vi "CSV - Add New Columns.vi"(8 "error in (no error)":errorcluster, 9 "LV Data Types":T1[](array[typedef]) format="%.0x", 10 "Headers":string[](array[string]), 11 "TableLogger_CSV_Actor in":refnum<class "TableLogger_CSV_Actor.lvclass">) -> (0 "error out":errorcluster, 3 "TableLogger_CSV_Actor out":refnum<class "TableLogger_CSV_Actor.lvclass">)   [LabVIEW 2014, in "TableLogger_CSV_Actor.lvlib" / "TableLogger_CSV_Actor.lvclass"]
uses:
  TableLogger_CSV_Actor.lvclass
  <userlib>/_OpenG.lib/lvdata/lvdata.llb/Type Descriptor Enumeration__ogtk.ctl
  TableLogger_CSV_Actor.lvclass/TableLogger_CSV_Actor.ctl
panel:
  # "Connector Pane"
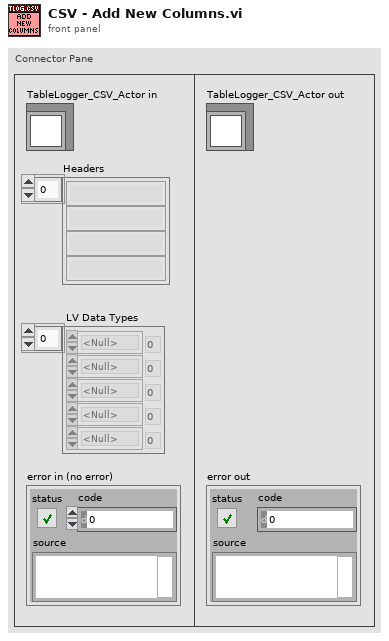
[diagram p1: front panel]
types:
  T1 = typedef "Type Descriptor Enumeration__ogtk.ctl" = enum8{"<Null>", "I8", "I16", "I32", "I64", "U8", "U16", "U32", "U64", "SGL", "DBL", "EXT", "CSG", "CDB", "CXT", "0x0F", "0x10", "0x11", "0x12", "0x13", "0x14", "Enum U8", "Enum U16", "Enum U32", "Enum U64", "SGL PQ", "DBL PQ", "EXT PQ", "CSG PQ", "CDB PQ", "CXT PQ", "0x1F", "0x20", "Boolean", "0x22", "0x23", "0x24", "0x25", "0x26", "0x27", "0x28", "0x29", "0x2A", "0x2B", "0x2C", "0x2D", "0x2E", "0x2F", "String", "0x31", "Path", "Pict", "0x34", "0x35", "0x36", "DAQ", "0x38", "0x39", "0x3A", "0x3B", "0x3C", "0x3D", "0x3E", "0x3F", "Array", "0x41", "0x42", "0x43", "0x44", "0x45", "0x46", "0x47", "0x48", "0x49", "0x4A", "0x4B", "0x4C", "0x4D", "0x4E", "0x4F", "Cluster", "0x51", "0x52", "Variant", "Waveform", "0x55", "0x56", "0x57", "0x58", "0x59", "0x5A", "0x5B", "0x5C", "0x5D", "0x5E", "0x5F", "0x60", "0x61", "0x62", "0x63", "0x64", "0x65", "0x66", "0x67", "0x68", "0x69", "0x6A", "0x6B", "0x6C", "0x6D", "0x6E", "0x6F", "Refnum"}
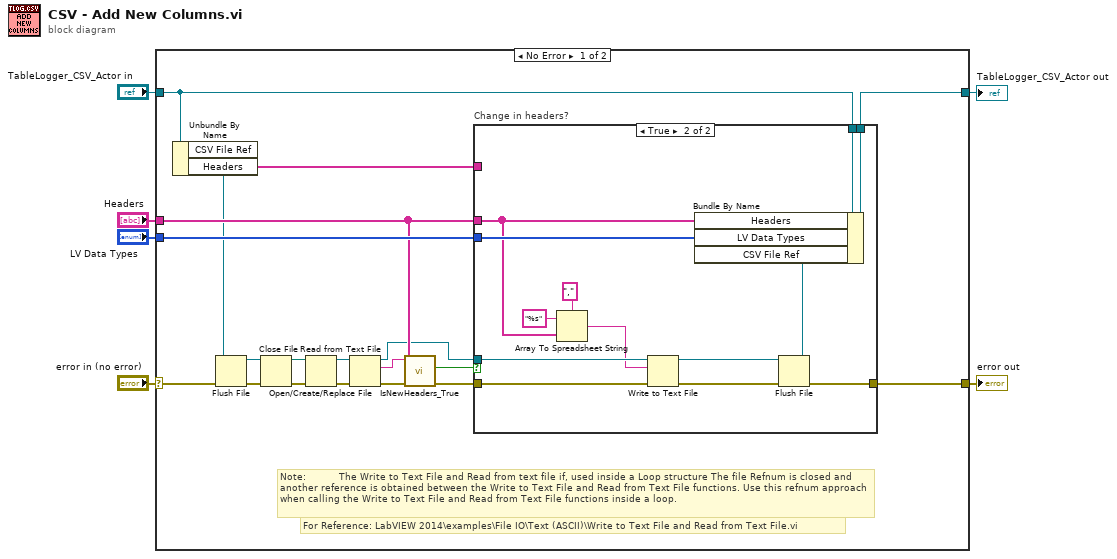
[diagram p0: block diagram]
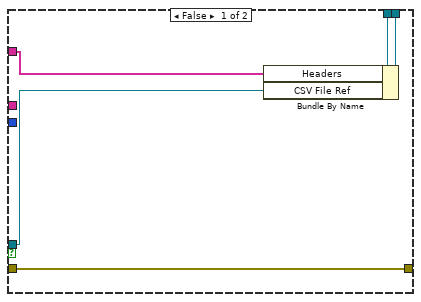
[diagram p2: hidden frame]
diagram:
  n1 = case shown="No Error" "error in (no error)" {
    selector: "error in (no error)" -> [w21 w44]
    tunnel: [w25 w45] -> w6
    tunnel: "Headers" -> [w19 _]
    tunnel: "LV Data Types" -> [w22 _]
    tunnel: [w23 w44] -> w2
    tunnel: "TableLogger_CSV_Actor in" -> [w24 w45]
    frame No Error {
      # "For Reference: LabVIEW 2014\\examples\\File IO\\Text (ASCII)\\Write to Text File and Read from Text File.vi"
      # "Note:           The Write to Text File and Read from text file if, used inside a Loop structure The file Refnum is closed and another reference is obtained between the Write to Text File and Read from Text File functions. Use this refnum approach when calling the Write to Text File and Read from Text File functions inside a loop."
      n2 = Unbundle By Name(w24) -> ("CSV File Ref"=w18:refnum<file>, "Headers"=w8:string[])
      n3 = Flush File(refnum=w18, error in=w21) -> (refnum out=w12:refnum<file>, error out=w10:errorcluster)
      n4 = Close File(refnum=w12, error in=w10) -> (path=w14:path, error out=w13:errorcluster)
      n5 = Open/Create/Replace File(file path (use dialog)=w14, error in=w13) -> (refnum out=w11:refnum<file>, error out=w9:errorcluster)  [unwired: 4 in, 1 out]
      n6 = Read from Text File(file (use dialog)=w11, error in=w9) -> (refnum out=w15:refnum<file>, text=w7:string, error out=w17:errorcluster)  [unwired: 2 in, 1 out]
      n7 = call "IsNewHeaders_True.vi"("error in"=w17, "Headers"=w19, "Data"=w7) -> ("error out"=w16:errorcluster, "Different Header?"=w20:bool)  [unwired: 6 in, 1 out]
      n8 = case "Change in headers?" shown="True" w20 {
        tunnel: [w28 w43] -> w25
        tunnel: w24 -> [w29 w42]
        tunnel: w16 -> [w30 w35]
        tunnel: [w30 w38] -> w23
        tunnel: w22 -> [_ w41]
        tunnel: w19 -> [_ w34]
        tunnel: w15 -> [w27 w36]
        tunnel: w8 -> [w26 _]
        frame False {
          n9 = Bundle By Name(cluster=w29, "Headers"=w26, "CSV File Ref"=w27) -> (w28:refnum<class "TableLogger_CSV_Actor.lvclass">)
        }
        frame True {
          n10 = Array To Spreadsheet String(delimiter (Tab)=",", array=w34, 3:"%s" ("format string")) -> (spreadsheet string=w33:string)
          n11 = Write to Text File(file (use dialog)=w36, text=w33, error in=w35) -> (refnum out=w40:refnum<file>, error out=w39:errorcluster)  [unwired: 1 in, 1 out]
          n12 = Flush File(refnum=w40, error in=w39) -> (refnum out=w37:refnum<file>, error out=w38:errorcluster)
          n13 = Bundle By Name(cluster=w42, "Headers"=w34, "LV Data Types"=w41, "CSV File Ref"=w37) -> (w43:refnum<class "TableLogger_CSV_Actor.lvclass">)
        }
      }
    }
    frame Error {
    }
  }
  "TableLogger_CSV_Actor out" <- w6
  "error out" <- w2
